vi "Capture@CoordSet(Org+2Edge)__Parameter.vi"(1 "ParamterIn":string) -> (0 "ParamterOut":string)   [LabVIEW 2019]
panel:
  in  "Org":string(combo)
  in  "YEdge":string(combo)
  in  "XEdge":string(combo)
  in  "CamName":string(combo)
  in  "Confirm":bool
  # "Capture@CoordSet $Capture,$Org,$XEdge,$YEdge\nOrg,Xedge,Yedge\nOrg[0]=O1\nXedge[0]=X1,Xedge[1]=X2\nYedge[0]=Y1,Yedge[1]=Y2"
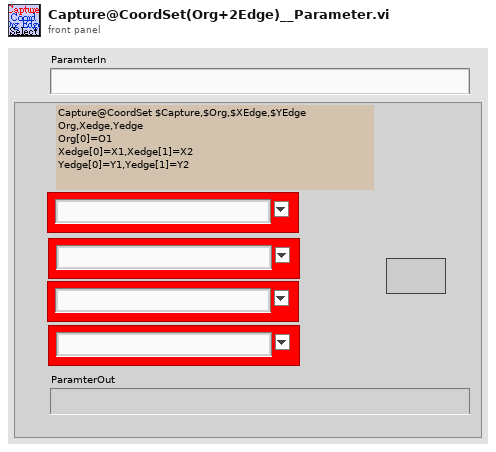
[diagram p1: front panel]
types:
  T1 = enum16{"Get", "UpdatePointS", "Init", "UpdateIndex", "GetCurrent&Index+1", "GetWithIndex", "ChkLast", "GetCurrent"}
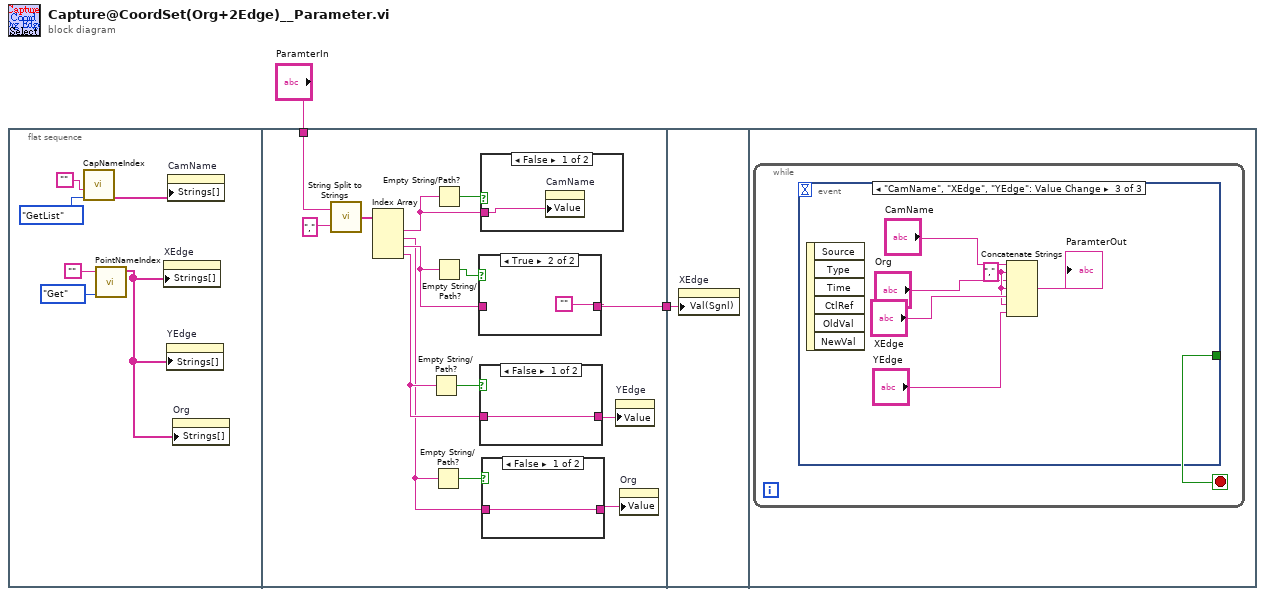
[diagram p0: block diagram]
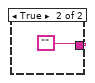
[diagram p2: hidden frame]
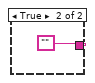
[diagram p3: hidden frame]
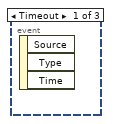
[diagram p6: hidden frame]
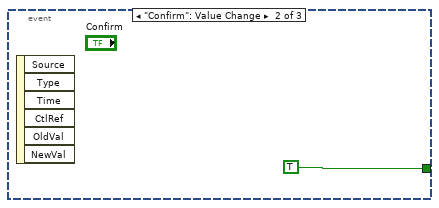
[diagram p7: hidden frame]
diagram:
  n1 = flat-sequence {
    tunnel: "ParamterIn" -> [w20]
    tunnel: [w16] -> w1
    tunnel: w1 -> [w30]
    frame #0 {
      n2 = call "CapNameIndex.vi"("OP"=enum16{"AddCam", "GetIndex", "Init", "GetList"}."GetList", "CamName"="") -> ("DeviceList"=w7:string[])  [unwired: 2 in, 3 out]
      n3 = call "PointNameIndex.vi"("OP"=T1."Get", "PointName"="") -> ("PointNameList"=w3:string[])  [unwired: 4 in, 5 out]
      n4 = property on="XEdge" class="CmbBox"("Strings[]"=w3) -> ()  [unwired: 2 in, 2 out]
      n5 = property on="YEdge" class="CmbBox"("Strings[]"=w3) -> ()  [unwired: 2 in, 2 out]
      n6 = property on="CamName" class="CmbBox"("Strings[]"=w7) -> ()  [unwired: 2 in, 2 out]
      n7 = property on="Org" class="CmbBox"("Strings[]"=w3) -> ()  [unwired: 2 in, 2 out]
    }
    frame #1 {
      n8 = call "String Split to Strings.vi"("search string/char (-)"=",", "String"=w20) -> ("Array"=w22:string[])
      n9 = Index Array(array=w22) -> (element #1=w18:string, element #2=w10:string, element #3=w12:string, element #4=w13:string)  [unwired: 4 in]
      n10 = Empty String/Path?(string/path=w13) -> (empty?=w15:bool)
      n11 = Empty String/Path?(string/path=w10) -> (empty?=w11:bool)
      n12 = Empty String/Path?(string/path=w18) -> (empty?=w19:bool)
      n13 = Empty String/Path?(string/path=w12) -> (empty?=w17:bool)
      n14 = case shown="True" w17 {
        tunnel: [w27 ""] -> w16
        tunnel: w12 -> [w27 _]
        frame False {
        }
        frame True {
        }
      }
      n15 = case shown="False" w15 {
        tunnel: [w25 ""] -> w14
        tunnel: w13 -> [w25 _]
        frame False {
        }
        frame True {
        }
      }
      n16 = case shown="False" w19 {
        tunnel: w18 -> [w29 _]
        frame False {
          n17 = property on="CamName" class="CmbBox"("Value"=w29) -> ()  [unwired: 2 in, 2 out]
        }
        frame True {
        }
      }
      n18 = case shown="False" w11 {
        tunnel: [w23 ""] -> w9
        tunnel: w10 -> [w23 _]
        frame False {
        }
        frame True {
        }
      }
      n19 = property on="YEdge" class="CmbBox"("Value"=w14) -> ()  [unwired: 2 in, 2 out]
      n20 = property on="Org" class="CmbBox"("Value"=w9) -> ()  [unwired: 2 in, 2 out]
    }
    frame #2 {
      n21 = property on="XEdge" class="CmbBox"("Val(Sgnl)"=w30) -> ()  [unwired: 2 in, 2 out]
    }
    frame #3 {
      n22 = while {
        stop <- w31 stop-if-true
        n23 = event shown="[2] \"CamName\", \"XEdge\", \"YEdge\": Value Change" {
          selector: _ -> [_ _ _]
          dyn-events: _ -> [_ _ _]
          timeout: _ -> [_ _ _]
          tunnel: [_ TRUE _] -> w31
          event Timeout {
            n24 = event-data() -> ()  [unwired: 1 in, 3 out]
          }
          event "Confirm": Value Change {
            n25 = event-data() -> ()  [unwired: 1 in, 6 out]
          }
          event "CamName", "XEdge", "YEdge": Value Change {
            w34 = "," ("string")
            n26 = event-data() -> ()  [unwired: 1 in, 6 out]
            n27 = Concatenate Strings("CamName", w34, "Org", w34, "XEdge", w34, "YEdge") -> (→"ParamterOut":string)
          }
        }
      }
    }
  }
